vi "Evaluate Boolean Evaluation Trigger.vi"(8 "error in (no error)":errorcluster, 10 "Trigger Data":dbl[](array[numeric]), 11 "Boolean Evaluation Trigger in":refnum<class "Boolean Evaluation Trigger.lvclass">) -> (0 "error out":errorcluster, 2 "Trigger":bool, 3 "Boolean Evaluation Trigger out":refnum<class "Boolean Evaluation Trigger.lvclass">)   [LabVIEW 2015, in "Boolean Evaluation Trigger.lvclass"]
uses:
  Boolean Evaluation Trigger.lvclass
  Boolean Evaluation Trigger.lvclass/Boolean Evaluation Trigger.ctl
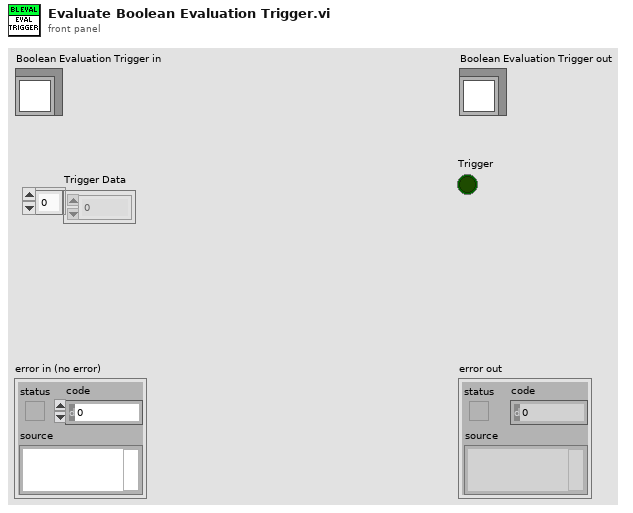
[diagram p1: front panel]
types:
  T1 = typedef "Boolean Evaluation Trigger.lvclass/Operand.ctl" = enum16{"==", "!=", "<", "<=", ">", ">="}
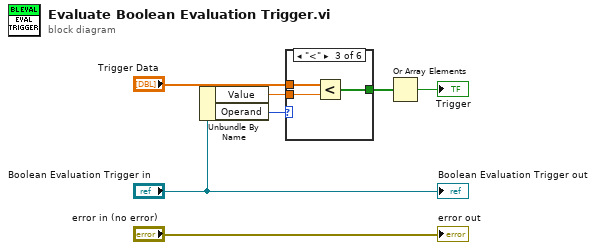
[diagram p0: block diagram]
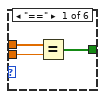
[diagram p2: hidden frame]
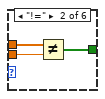
[diagram p3: hidden frame]
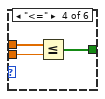
[diagram p4: hidden frame]
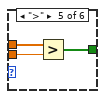
[diagram p5: hidden frame]
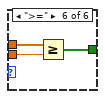
[diagram p6: hidden frame]
diagram:
  n1 = Unbundle By Name("Boolean Evaluation Trigger in") -> ("Value"=w3:dbl, "Operand"=w7:T1)
  n2 = case shown="\"<\"" w7 {
    tunnel: "Trigger Data" -> [w9 w12 w15 w18 w21 w24]
    tunnel: w3 -> [w10 w13 w16 w19 w22 w25]
    tunnel: [w8 w11 w14 w17 w20 w23] -> w2
    frame "==" {
      n3 = Equal?(x=w9, y=w10) -> (x = y?=w8:bool[])
    }
    frame "!=" {
      n4 = Not Equal?(x=w12, y=w13) -> (x != y?=w11:bool[])
    }
    frame "<" {
      n5 = Less?(x=w15, y=w16) -> (x < y?=w14:bool[])
    }
    frame "<=" {
      n6 = Less Or Equal?(x=w18, y=w19) -> (x <= y?=w17:bool[])
    }
    frame ">" {
      n7 = Greater?(x=w21, y=w22) -> (0:w20:bool[])
    }
    frame ">=" {
      n8 = Greater Or Equal?(x=w24, y=w25) -> (x >= y?=w23:bool[])
    }
  }
  n9 = Or Array Elements(Boolean array=w2) -> (logical OR=→"Trigger":bool)
  "error out" <- "error in (no error)"
  "Boolean Evaluation Trigger out" <- "Boolean Evaluation Trigger in"
